vi "Write and Read Multiple Holding Registers.vi"(4 "read count":u16, 6 "read starting address":u16, 8 "error in":errorcluster, 9 "write values":u16[](array[numeric]), 10 "write starting address":u16, 11 "Modbus instance in":refnum<class "Modbus Slave.lvclass">) -> (0 "error out":errorcluster, 1 "read values":u16[](array[numeric]), 3 "Modbus instance out":refnum<class "Modbus Slave.lvclass">)   [LabVIEW 2012, in "Modbus Slave.lvclass"]
doc: "Writes and reads the values of multiple register values in series. The <b>write values</b> are inserted starting at <b>write starting address</b> and the returned <b>read values</b> consists of <b>read count</b> holding registers starting at <b>read starting address</b>."
uses:
  Modbus Slave.lvclass
  Modbus Slave.lvclass/Modbus Slave.ctl
  Data Model/Device Data Model.lvclass
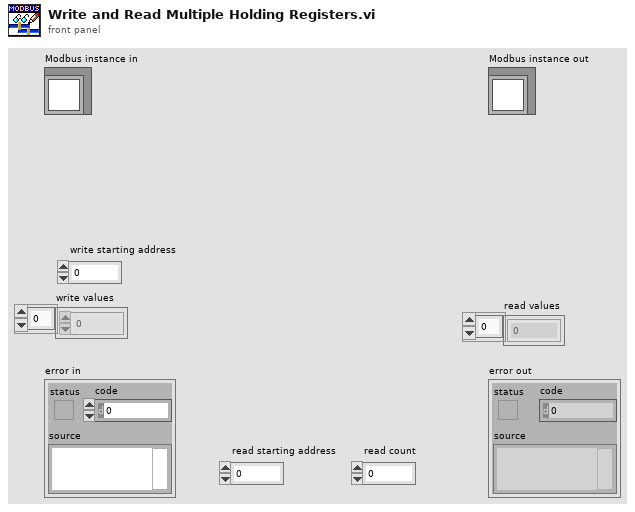
[diagram p1: front panel]
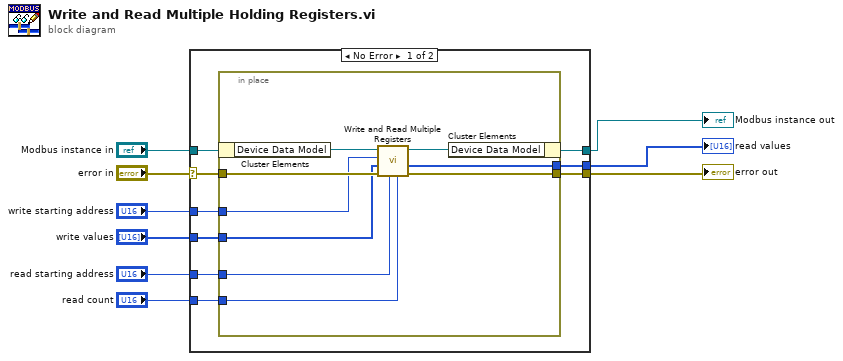
[diagram p0: block diagram]
diagram:
  n1 = case shown="No Error" "error in" {
    selector: "error in" -> [w16 w29]
    tunnel: [w17 w29] -> w1
    tunnel: "Modbus instance in" -> [w18 w28]
    tunnel: [w15 w28] -> w8
    tunnel: [w14 _] -> w7
    tunnel: "read starting address" -> [w13 _]
    tunnel: "read count" -> [w12 _]
    tunnel: "write starting address" -> [w11 _]
    tunnel: "write values" -> [w10 _]
    frame No Error {
      n2 = in-place {
        in-place-border: [w27] -> w17
        in-place-border: w16 -> [w26]
        in-place-border: [w23] -> w14
        in-place-border: w13 -> [w22]
        in-place-border: w12 -> [w21]
        in-place-border: w11 -> [w20]
        in-place-border: w10 -> [w19]
        n3 = in-place-cluster #1(w18) -> ("Device Data Model"=w24:refnum<class "Device Data Model.lvclass">)
        n4 = call-dynamic "Write and Read Multiple Registers.vi"("read count"=w21, "read starting address"=w22, "error in"=w26, "write values"=w19, "write starting address"=w20, "device data model in"=w24) -> ("error out"=w27:errorcluster, "read values"=w23:u16[], "device data model out"=w25:refnum<class "Device Data Model.lvclass">)  [unwired: 3 in]
        n5 = in-place-cluster #1("Device Data Model"=w25) -> (w15:refnum<class "Modbus Slave.lvclass">)
      }
    }
    frame Error {
    }
  }
  "error out" <- w1
  "Modbus instance out" <- w8
  "read values" <- w7
